vi "Logfile_Data_Line.vi"(2 "System Monitor Cluster":T1={"Time"=[], "LI1CH1"=[], "LI1CH2"=[], "LI2CH1"=[], "LI2CH2"=[], "LI3CH1"=[], "LI3CH2"=[], "Field"=[], "Temperature"=[], "Temperature 2"=[], "Temperatrue 3"=[], "Nitrogen_Level"=[], "Helium_Level"=[], "Heater_LS370"=[], "Sorb_Heater"=[], "Still_Heater"=[], "Capacity"=[], "Loss"=[], "Magnet_Temperature"=[], "Lambda_Pressure"=[], "Lambda_Needle_Valve"=[], "LS370-CH1-T"=[], "LS370-CH2-T"=[], "LS370-CH3-T"=[], "LS370-CH4-T"=[], "LS370-TC-T"=[], "LS370-CH1-R"=[], "LS370-CH2-R"=[], "LS370-CH3-R"=[], "LS370-CH4-R"=[], "LS370-TC-R"=[], "LS372-CH1-T"=[], "LS372-CH2-T"=[], "LS372-CH3-T"=[], "LS372-CH4-T"=[], "LS372-CH5-T"=[], "LS372-CH6-T"=[], "LS372-CH1-R"=[], "LS372-CH2-R"=[], "LS372-CH3-R"=[], "LS372-CH4-R"=[], "LS372-CH5-R"=[], "LS372-CH6-R"=[], "Nada"=[nan], "Keithley_Res"=[], "Keithley_Current"=[], "VTI_Heater"=[], "VTI_Needle Valve"=[], "LS340_Heater"=[], "Keithley_6221_Amplitude"=[], "Keithley_6221_Frequency"=[], "Condense_Pressure"=[], "Still_Pressure"=[], "FP_Out_Pressure"=[], "Dump_Pressure"=[], "V1"=[], "V2"=[], "V4"=[], "V5"=[], "V9"=[], "Forepump"=[], "Compressor"=[], "Keihtley_6221_Offset"=[], "BoxTemp"=[], "By"=[], "Bz"=[], "Phi"=[], "heater-recond (%)"=[], "Dewar Pressure "=[], "JT-Control-Setpoint"=[], "LS350 T1"=[], "LS350 T2"=[], "LS350 T3"=[], "LS350 T4"=[], "LS350 R1"=[], "LS350 R2"=[], "LS350 R3"=[], "LS350 R4"=[]}) -> (0 "Data Line":string)   [LabVIEW 2016]
uses:
  Global/Global Variables/System Monitor Cluster.ctl
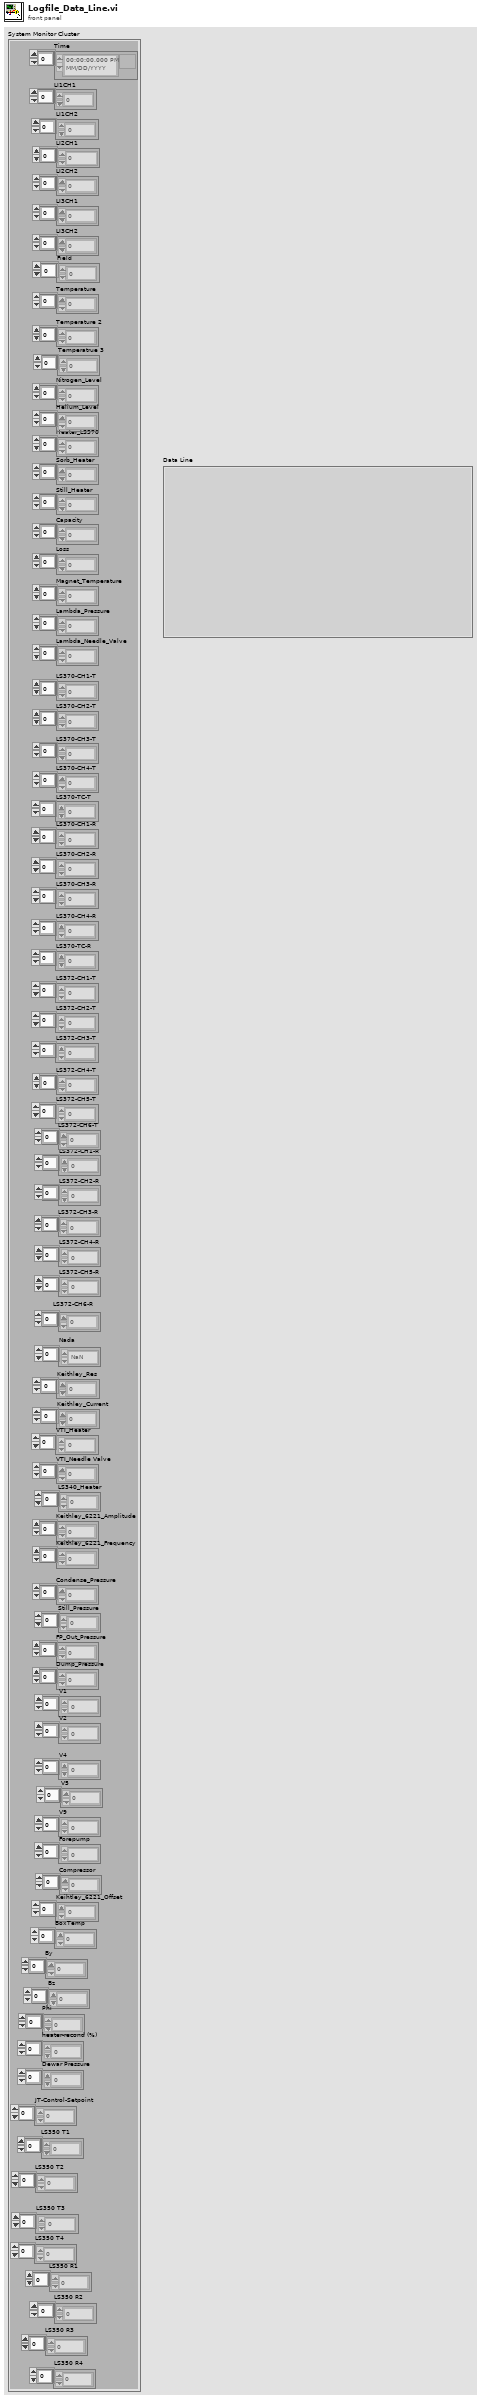
[diagram p1: front panel]
types:
  T1 = typedef "System Monitor Cluster.ctl" = cluster{"Time":timestamp[], "LI1CH1":dbl[], "LI1CH2":dbl[], "LI2CH1":dbl[], "LI2CH2":dbl[], "LI3CH1":dbl[], "LI3CH2":dbl[], "Field":dbl[], "Temperature":dbl[], "Temperature 2":dbl[], "Temperatrue 3":dbl[], "Nitrogen_Level":dbl[], "Helium_Level":dbl[], "Heater_LS370":dbl[], "Sorb_Heater":dbl[], "Still_Heater":dbl[], "Capacity":dbl[], "Loss":dbl[], "Magnet_Temperature":dbl[], "Lambda_Pressure":dbl[], "Lambda_Needle_Valve":dbl[], "LS370-CH1-T":dbl[], "LS370-CH2-T":dbl[], "LS370-CH3-T":dbl[], "LS370-CH4-T":dbl[], "LS370-TC-T":dbl[], "LS370-CH1-R":dbl[], "LS370-CH2-R":dbl[], "LS370-CH3-R":dbl[], "LS370-CH4-R":dbl[], "LS370-TC-R":dbl[], "LS372-CH1-T":dbl[], "LS372-CH2-T":dbl[], "LS372-CH3-T":dbl[], "LS372-CH4-T":dbl[], "LS372-CH5-T":dbl[], "LS372-CH6-T":dbl[], "LS372-CH1-R":dbl[], "LS372-CH2-R":dbl[], "LS372-CH3-R":dbl[], "LS372-CH4-R":dbl[], "LS372-CH5-R":dbl[], "LS372-CH6-R":dbl[], "Nada":dbl[], "Keithley_Res":dbl[], "Keithley_Current":dbl[], "VTI_Heater":dbl[], "VTI_Needle Valve":dbl[], "LS340_Heater":dbl[], "Keithley_6221_Amplitude":dbl[], "Keithley_6221_Frequency":dbl[], "Condense_Pressure":dbl[], "Still_Pressure":dbl[], "FP_Out_Pressure":dbl[], "Dump_Pressure":dbl[], "V1":dbl[], "V2":dbl[], "V4":dbl[], "V5":dbl[], "V9":dbl[], "Forepump":dbl[], "Compressor":dbl[], "Keihtley_6221_Offset":dbl[], "BoxTemp":dbl[], "By":dbl[], "Bz":dbl[], "Phi":dbl[], "heater-recond (%)":dbl[], "Dewar Pressure ":dbl[], "JT-Control-Setpoint":dbl[], "LS350 T1":dbl[], "LS350 T2":dbl[], "LS350 T3":dbl[], "LS350 T4":dbl[], "LS350 R1":dbl[], "LS350 R2":dbl[], "LS350 R3":dbl[], "LS350 R4":dbl[]}
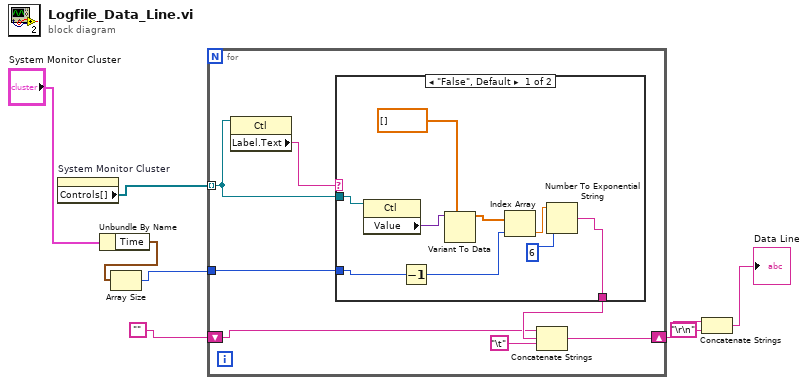
[diagram p0: block diagram]
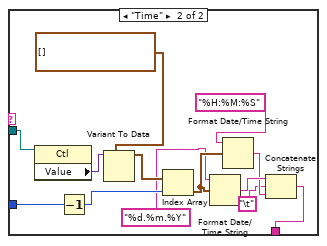
[diagram p2: hidden frame]
diagram:
  n1 = property on="System Monitor Cluster" class="Clust (strict)"() -> ("Controls[]"=w8:refnum<vi>[])  [unwired: 2 in, 2 out]
  n2 = Unbundle By Name("System Monitor Cluster") -> ("Time"=w2:timestamp[])
  n3 = Array Size(array=w2) -> (size(s)=w1:i32)
  n4 = for {
    tunnel: w8 -> [w15] mode=indexing
    shift-right: [w10] -> w6
    shift-left: "" -> [w11]
    tunnel: w1 -> [w9]
    n5 = property class="Ctl"(reference=w15) -> ("Label.Text"=w14:string)  [unwired: 1 in, 2 out]
    n6 = case shown="\"False\", Default" w14 {
      tunnel: w15 -> [w24 w37]
      tunnel: [w16 w31] -> w13
      tunnel: w9 -> [w20 w30]
      frame "False", Default {
        n7 = property class="Ctl"(reference=w24) -> ("Value"=w22:variant)  [unwired: 1 in, 2 out]
        n8 = Decrement(x=w20) -> (x-1=w19:i32)
        n9 = Variant To Data(type=dbl[] [], Variant=w22) -> (data=w21:dbl[])  [unwired: 1 in, 1 out]
        n10 = Index Array(array=w21, index=w19) -> (element=w18:dbl)
        n11 = Number To Exponential String(number=w18, 3:6) -> (E-format string=w16:string)  [unwired: 2 in]
      }
      frame "Time" {
        n12 = property class="Ctl"(reference=w37) -> ("Value"=w35:variant)  [unwired: 1 in, 2 out]
        n13 = Decrement(x=w30) -> (x-1=w29:i32)
        n14 = Variant To Data(type=timestamp[] [], Variant=w35) -> (data=w34:timestamp[])  [unwired: 1 in, 1 out]
        n15 = Index Array(array=w34, index=w29) -> (element=w32:timestamp)
        n16 = Format Date/Time String(time format string (%c)="%d.%m.%Y", seconds (now)=w32) -> (date/time string=w27:string)  [unwired: 1 in]
        n17 = Format Date/Time String(time format string (%c)="%H:%M:%S", seconds (now)=w32) -> (date/time string=w26:string)  [unwired: 1 in]
        n18 = Concatenate Strings(w27, "\t", w26) -> (w31:string)
      }
    }
    n19 = Concatenate Strings(w11, w13, "\t") -> (w10:string)
  }
  n20 = Concatenate Strings(w6, "\r\n") -> (→"Data Line":string)
